vi "Get Flex Channel.vi"(6 "User App":refnum<vi>, 7 "app":refnum<vi>, 10 "Item Path":path, 11 "Element Type":variant) -> (3 "Channel Type":variant)   [LabVIEW 2022 SP3, in "FlexBlocks Support.lvlib"]
uses:
  FlexBlocks Support.lvlib
  <vilib>/Utility/Data Type/Type Definitions/Data Type.ctl
  <vilib>/Utility/Data Type/Type Definitions/Type Definition Info.ctl
  <vilib>/Utility/Data Type/NI_Data Type.lvlib
panel:
  out "type definition path 3":path
  out "Channel Info Error":errorcluster
  out "type 2":T1
  out "name 2":string
  out "type definition 2":bool
  out "type definition info 2":T2
  out "type definition path 2":path
  out "type definition path":path
  out "type definition info":T2
  out "type definition":bool
  out "name":string
  out "type":T1
  out "error out":errorcluster
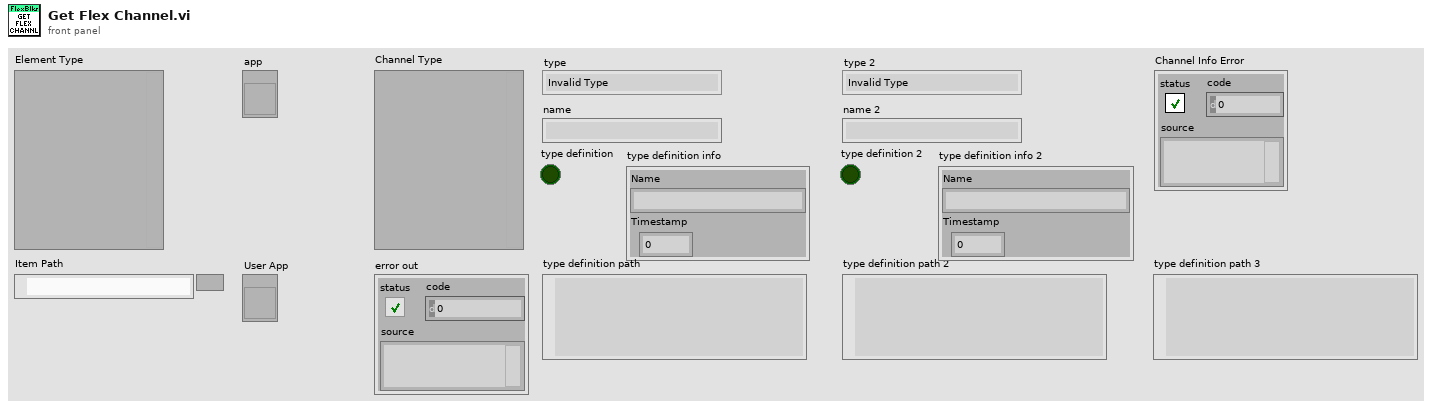
[diagram p1: front panel]
types:
  T1 = typedef "NI_Data Type.lvlib/Data Type.ctl" = enum8{"Invalid Type", "Void", "I8", "I16", "I32", "I64", "U8", "U16", "U32", "U64", "Single Float", "Double Float", "Extended Float", "Single Complex", "Double Complex", "Extended Complex", "Enum U8", "Enum U16", "Enum U32", "Enum U64", "Single Float With Unit", "Double Float With Unit", "Extended Float With Unit", "Single Complex with Unit", "Double Complex with Unit", "Extended Complex with Unit", "Boolean", "String", "Path", "Picture", "Tag", "Array", "Cluster", "Variant", "LV Variant", "Waveform", "Timestamp", "Digital Waveform", "Digital Data", "ExpressData", "Refnum", "External Data", "VI", "Poly VI", "LabVIEW Class Instance", "Fixed Point", "Set Collection", "Map Collection"}
  T2 = typedef "NI_Data Type.lvlib/Type Definition Info.ctl" = cluster{"Name":string, "Timestamp":u32}
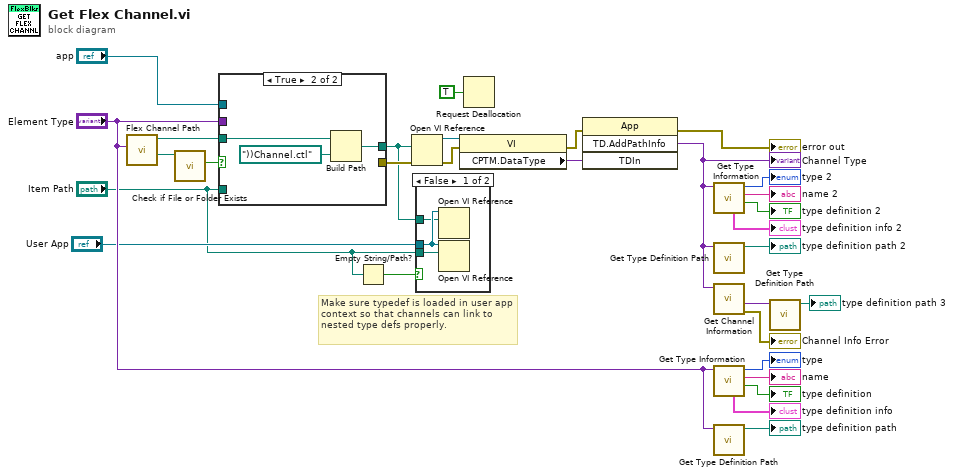
[diagram p0: block diagram]
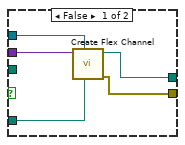
[diagram p3: hidden frame]
diagram:
  # "Make sure typedef is loaded in user app context so that channels can link to nested type defs properly."
  n1 = call "Flex Channel Path.vi"("Variant"="Element Type") -> ("Channel Library Path"=w16:path, "Channel Folder Path"=w15:path)  [unwired: 9 in]
  n2 = call <vilib>:"Check if File or Folder Exists.vi"("path"=w16) -> ("file or folder exists?"=w17:bool)  [unwired: 8 in, 2 out]
  n3 = case shown="True" w17 {
    tunnel: "Element Type" -> [w35 _]
    tunnel: "app" -> [w34 _]
    tunnel: "Item Path" -> [w33 _]
    tunnel: w15 -> [_ w38]
    tunnel: [w32 w36] -> w5
    tunnel: [w31 _] -> w13
    frame False {
      n4 = call "Create Flex Channel.vi"("Item Path"=w33, "app"=w34, "Element Type"=w35) -> ("error IO"=w31:errorcluster, "Channel Control Path"=w32:path)  [unwired: 7 in]
    }
    frame True {
      n5 = Build Path(base path=w38, name or relative path=path "))Channel.ctl") -> (appended path=w36:path)
    }
  }
  n6 = Empty String/Path?(string/path="Item Path") -> (empty?=w6:bool)
  n7 = Open VI Reference(vi path=w5, error in (no error)=w13) -> (vi reference=w18:refnum<vi>, error out=w19:errorcluster)  [unwired: 4 in]
  n8 = case shown="False" w6 {
    tunnel: "User App" -> [w40 _]
    tunnel: "Item Path" -> [w41 _]
    tunnel: w5 -> [w39 _]
    frame False {
      n9 = Open VI Reference(application reference (local)=w40, vi path=w39) -> ()  [unwired: 4 in, 2 out]
      n10 = Open VI Reference(application reference (local)=w40, vi path=w41) -> ()  [unwired: 4 in, 2 out]
    }
    frame True {
    }
  }
  n11 = property class="VI"(reference=w18, error in=w19) -> (error out=w3:errorcluster, "CPTM.DataType"=w4:variant)  [unwired: 1 out]
  n12 = Request Deallocation(TRUE ("flag")) -> ()
  n13 = invoke class="App" method="TD.AddPathInfo"(error in=w3, "TDIn"=w4) -> (error out=→"error out":errorcluster, "TD.AddPathInfo"=w2:variant)  [unwired: 2 in, 2 out]
  "Channel Type" <- w2
  n14 = call <vilib>:"Get Type Information.vi"("variant"=w2) -> ("type definition"=→"type definition 2":bool, "name"=→"name 2":string, "type"=→"type 2":T1, "type definition info"=→"type definition info 2":T2)  [unwired: 6 in, 1 out]
  n15 = call <vilib>:"Get Type Definition Path.vi"("variant"=w2) -> ("type definition path"=→"type definition path 2":path)  [unwired: 9 in, 1 out]
  n16 = call <vilib>:"Get Channel Information.vi"("variant"=w2) -> ("error out"=→"Channel Info Error":errorcluster, "element type"=w11:variant)  [unwired: 6 in, 3 out]
  n17 = call <vilib>:"Get Type Information.vi"("variant"="Element Type") -> ("type definition"=→"type definition":bool, "name"=→"name":string, "type"=→"type":T1, "type definition info"=→"type definition info":T2)  [unwired: 6 in, 1 out]
  n18 = call <vilib>:"Get Type Definition Path.vi"("variant"="Element Type") -> ("type definition path"=→"type definition path":path)  [unwired: 9 in, 1 out]
  n19 = call <vilib>:"Get Type Definition Path.vi"("variant"=w11) -> ("type definition path"=→"type definition path 3":path)  [unwired: 9 in, 1 out]
